vi "Triangular Egde Generator.vi"(8 "Sample values":dbl[](graph), 11 "Triangular edge":enum16{"Rising", "Falling"}(ring)=enum."Falling") -> (2 "Skew Triangular":dbl[](array[numeric]))   [LabVIEW 2014]
uses:
  <vilib>/imath/engines/lvmath2/RunTimeEngine/BuiltInFunctions/linramp/NIMS_linramp.vi
  <vilib>/imath/engines/lvmath2/RunTimeEngine/NodeEndStatement/NIMS_NodeEndStatement_Output.vi
  <instcachedir>/0/NIMS_NodeEndStatement_Output_53EC0D466D134D7ABD903AC30B43404B.lvgen/NIMS_NodeEndStatement_Output_53EC0D466D134D7ABD903AC30B43404B_005.vi
  <vilib>/imath/engines/lvmath2/RunTimeEngine/ErrorHandling/NIMS_Finalize Error.vi
  <vilib>/imath/engines/lvmath2/RunTimeEngine/ArithmeticOperatorToken/NIMS_ArithmeticOperator_times.vi
  <instcachedir>/0/NIMS_ArithmeticOperator_times_2EFF5B13FCA4492A81D59089AD809F54.lvgen/NIMS_ArithmeticOperator_times_2EFF5B13FCA4492A81D59089AD809F54_000.vi
  <vilib>/imath/engines/lvmath2/RunTimeEngine/BuiltInFunctions/max/1 input/NIMS_max(RV).vi
  <instcachedir>/0/NIMS_max(RV)_237633DB1D604D5BA7001287DF3C7957.lvgen/NIMS_max(RV)_237633DB1D604D5BA7001287DF3C7957_000.vi
  <vilib>/imathl/engines/lvmath/Functions/Error Handling/Create Error.vi
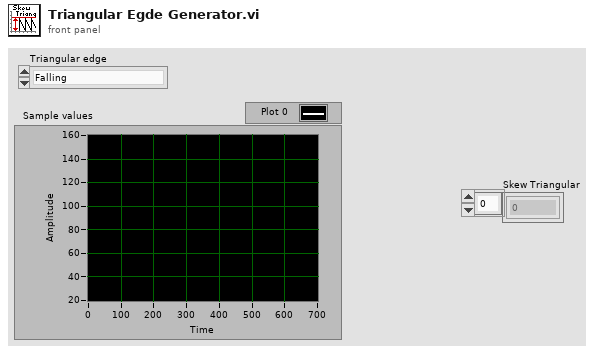
[diagram p1: front panel]
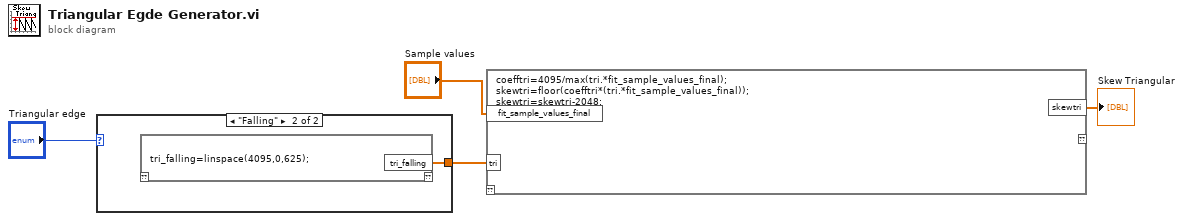
[diagram p0: block diagram]
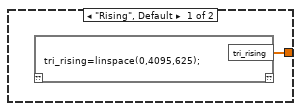
[diagram p2: hidden frame]
diagram:
  n1 = case shown="\"Falling\"" "Triangular edge" {
    tunnel: [w5 w25] -> w3
    frame "Rising", Default {
      n2 = mathscript code="tri_rising=linspace(0,4095,625);"() -> ("tri_rising"=w5:dbl[])  [unwired: 1 in, 1 out]
    }
    frame "Falling" {
      n3 = mathscript code="tri_falling=linspace(4095,0,625);"() -> ("tri_falling"=w25:dbl[])  [unwired: 1 in, 1 out]
    }
  }
  n4 = mathscript code="coefftri=4095/max(tri.*fit_sample_values_final);\nskewtri=floor(coefftri*(tri.*fit_sample_values_final));\nskewtri=skewtri-2048;"("tri"=w3, "fit_sample_values_final"="Sample values") -> ("skewtri"=→"Skew Triangular":dbl[])  [unwired: 1 in, 1 out]
